vi "NF LI56xx dvr ERRor.vi"(0 "VISA resource name":refnum<visa-resource-name>, 11 "error in (no error)":errorcluster caption="Error IN") -> (4 "VISA recource name copy":refnum<visa-resource-name>, 6 "ErrorNo":i32, 8 "Error":string, 15 "error out":errorcluster caption="Error OUT")   [LabVIEW 2019]
doc: "This VI queries the instrument for any errors in the instrument's error queue."
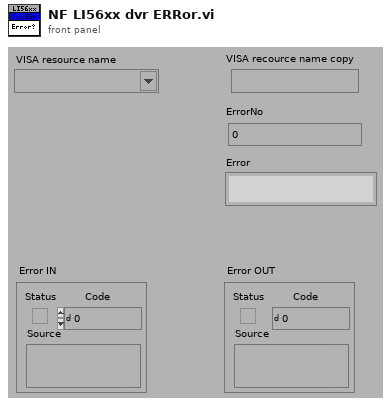
[diagram p1: front panel]
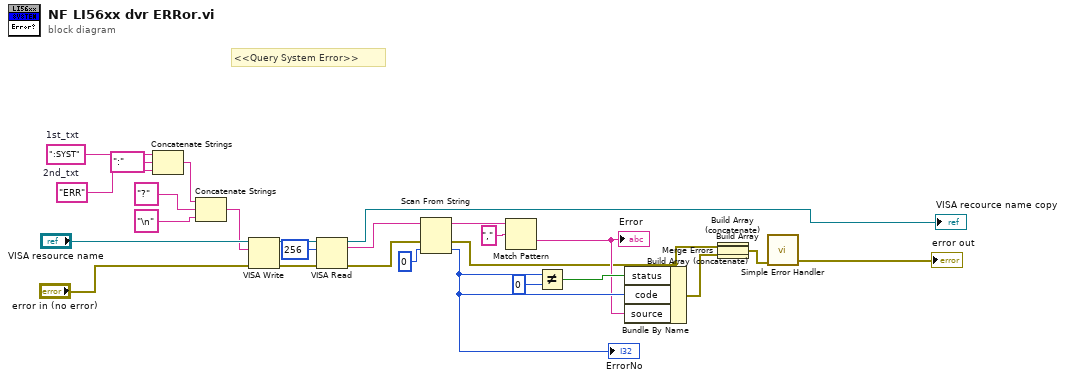
[diagram p0: block diagram]
diagram:
  w26 = "ERR"  # 2nd_txt
  w27 = ":SYST"  # 1st_txt
  # "<<Query System Error>>"
  n1 = Concatenate Strings(w27, ":" ("•¶Žš—ñ"), w26) -> (w25:string)
  n2 = Concatenate Strings(w25, "?" ("Œ`Ž®•¶Žš—ñ"), "\n" ("Œ`Ž®•¶Žš—ñ")) -> (w20:string)
  n3 = VISA Write(VISA resource name="VISA resource name", write buffer=w20, error in (no error)="error in (no error)") -> (VISA resource name out=w22:refnum<visa-resource-name>, error out=w23:errorcluster)  [unwired: 1 out]
  n4 = VISA Read(VISA resource name=w22, byte count=u32 256 ("バイトカウント（0）"), error in (no error)=w23) -> (VISA resource name out=→"VISA recource name copy":refnum<visa-resource-name>, read buffer=w14:string, error out=w18:errorcluster)  [unwired: 1 out]
  n5 = Scan From String(input string=w14, error in=w18, default 1=0 ("デフォルト1")) -> (remaining string=w16:string, error out=w8:errorcluster, output 1=w11:i32)  [unwired: 2 in, 1 out]
  "ErrorNo" <- w11
  n6 = Match Pattern(string=w16, regular expression="," ("³K\\»")) -> (after substring=w10:string)  [unwired: 4 out]
  "Error" <- w10
  n7 = Not Equal?(x=w11, y=0) -> (x != y?=w13:bool)
  n8 = Bundle By Name(cluster=w8, "status"=w13, "code"=w11, "source"=w10) -> (w7:errorcluster)
  n9 = Build Array(w8, w7) -> (w6:errorcluster[])
  n10 = Build Array (concatenate)(w6) -> (w5:errorcluster[])
  n11 = Build Array (concatenate)(w5) -> (w4:errorcluster[])
  n12 = Merge Errors(w4) -> (w9:errorcluster)
  n13 = call <vilib>:"Simple Error Handler.vi"("error in (no error)"=w9) -> ("error out"=→"error out":errorcluster)  [unwired: 1 in, 7 out]
